vi "Initialize Value Change Trigger.vi"(8 "error in (no error)":errorcluster, 11 "Value Change Trigger in":refnum<class "Value Change Trigger.lvclass">) -> (0 "error out":errorcluster, 3 "Value Change Trigger out":refnum<class "Value Change Trigger.lvclass">)   [LabVIEW 2012, in "Waveform Data Logger Engine.lvlib" / "Value Change Trigger.lvclass"]
uses:
  Value Change Trigger.lvclass
  Value Change Trigger.lvclass/Value Change Trigger.ctl
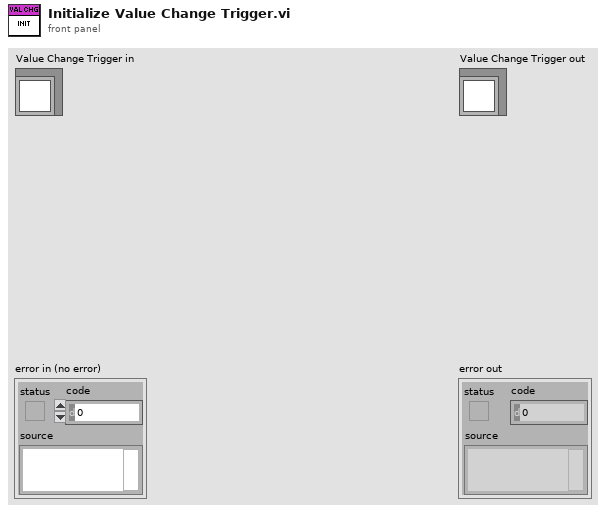
[diagram p1: front panel]
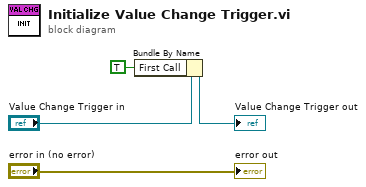
[diagram p0: block diagram]
diagram:
  n1 = Bundle By Name(cluster="Value Change Trigger in", "First Call"=TRUE) -> (→"Value Change Trigger out":refnum<class "Value Change Trigger.lvclass">)
  "error out" <- "error in (no error)"
